vi "FGV_Z_Array.vi"(8 "error in":errorcluster, 10 "Action":T1, 11 "Z_Array IN":dbl[](array[numeric])) -> (0 "error out":errorcluster, 2 "Z stack Size":u16, 3 "Z_Array OUT":dbl[](array[numeric]))   [LabVIEW 2026]
doc: "Functional Global Variable:\n- Write the value into the memory \nor\n- Read the value from the memory"
uses:
  TypeDef_FGV.ctl
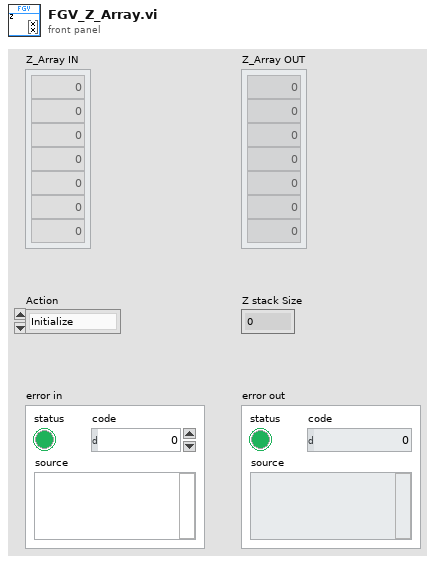
[diagram p1: front panel]
types:
  T1 = typedef "TypeDef_FGV.ctl" = enum16{"Initialize", "Write", "Read", "Read_File", "Write_to_File"}
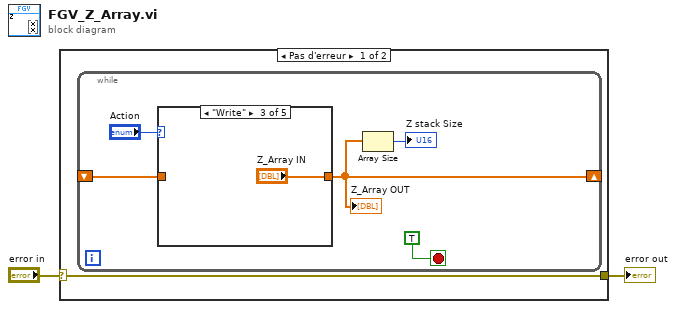
[diagram p0: block diagram]
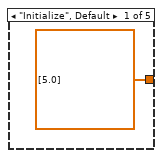
[diagram p2: hidden frame]
diagram:
  n1 = case shown="Pas d'erreur" "error in" {
    selector: "error in" -> [w3 w14]
    tunnel: [w3 w14] -> w1
    frame No Error {
      n2 = while {
        shift-right: [w4] -> _
        shift-left: _ -> [w6]
        stop <- TRUE stop-if-true
        n3 = case shown="\"Write\"" "Action" {
          tunnel: w6 -> [_ w10 _ w12 w13]
          tunnel: [dbl[] [5.0] ("Polar_Array IN") w10 "Z_Array IN" w12 w13] -> w4
          frame "Initialize", Default {
          }
          frame "Read" {
          }
          frame "Write" {
          }
          frame "Read_File" {
            # "A FAIRE"
          }
          frame "Write_to_File" {
            # "A Faire"
          }
        }
        "Z_Array OUT" <- w4
        n4 = Array Size(array=w4) -> (size(s)=→"Z stack Size":i32)
      }
    }
    frame Error {
    }
  }
  "error out" <- w1
